vi "Projection View.vi"(6 "Control Ref Queue":T1, 8 "error in (no error)":errorcluster, 11 "3D Plot.lvclass in":refnum<class "3D Plot.lvclass">) -> (0 "error out":errorcluster, 3 "3D Plot.lvclass out":refnum<class "3D Plot.lvclass">)   [LabVIEW 2020, in "3D Plot.lvclass"]
uses:
  3D Plot.lvclass
  3DMathPlot Ctrl Act Queue.ctl
  3DMathPlot Ctrl Act Cluster.ctl
  3DMathPlot State Class.ctl
  3D Plot.lvclass/3D Plot.ctl
  NI_3D Picture Control.lvlib
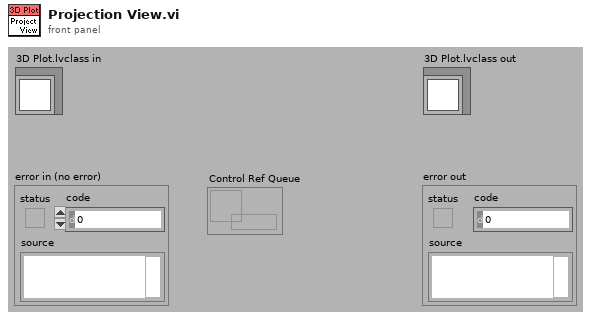
[diagram p1: front panel]
types:
  T1 = typedef "3DMathPlot Ctrl Act Queue.ctl" = refnum<queue>
  T2 = enum32{"Towards X-Y Plane", "Towards X-Z Plane", "Towards Y-Z Plane", "User Defined"}
  T3 = cluster{"View Latitude":sgl, "View Longitude":sgl, "View Distance":sgl}
  T4 = typedef "3DMathPlot Ctrl Act Cluster.ctl" = cluster{"3D Picture Control":refnum<vi>, "Render Window Refnum":refnum<vi>, "XY Graph":refnum<vi>, "Intensity Graph":refnum<vi>, "Color Legend Palette":refnum<vi>, "Projection Palette":refnum<vi>, "XControl  Ref":refnum<vi>, "Facade Ref":refnum<vi>, "Export Image Ref":refnum<vi>, "Clear Data Flag":bool, "Display State Change Class":T5}
  T5 = typedef "3DMathPlot State Class.ctl" = enum16{"Update All Objects (Undo)", "Update Light Object Only", "Update Axis Object Only", "Update Plot Object Only", "Update Cursor Object Only", "Update Axis Plot Cursor Objects", "No Update"}
  T6 = enum16{"None", "Spherical", "Flying", "Oriented"}
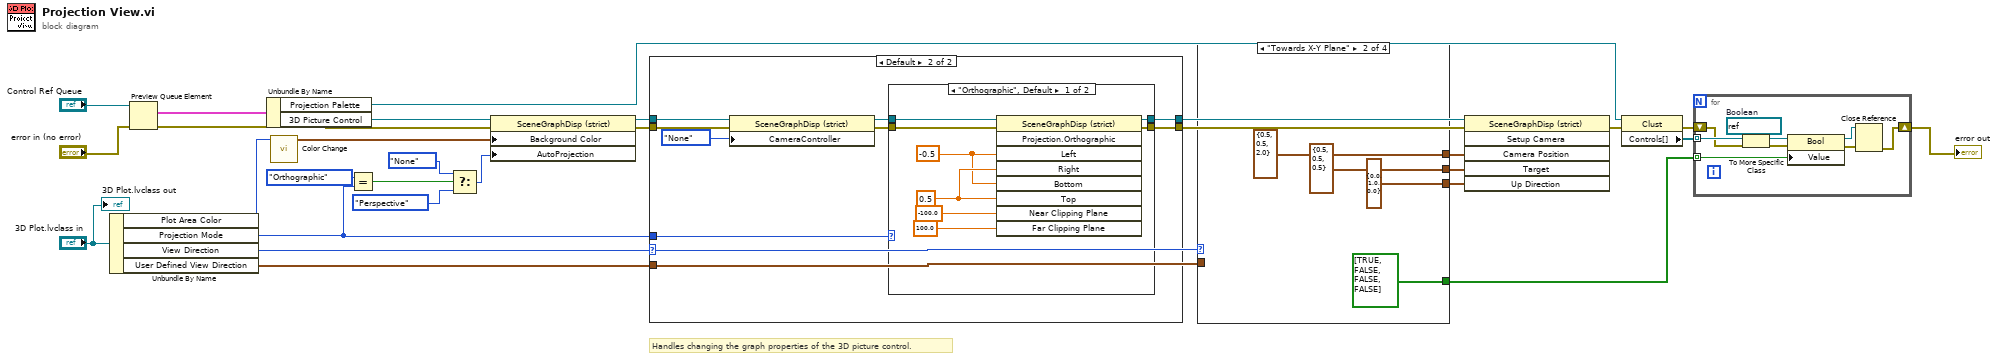
[diagram p0: block diagram]
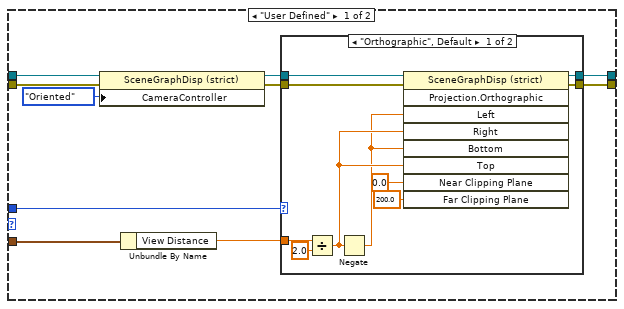
[diagram p2: hidden frame]
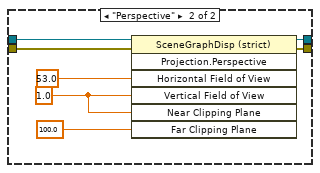
[diagram p4: hidden frame]
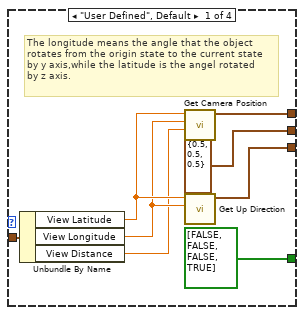
[diagram p5: hidden frame]
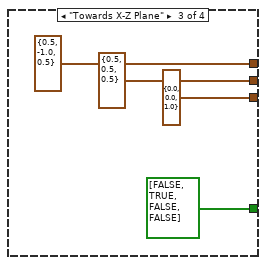
[diagram p6: hidden frame]
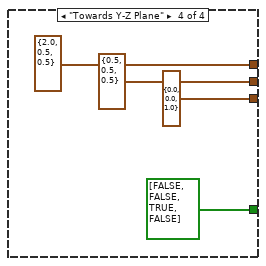
[diagram p7: hidden frame]
diagram:
  # "Handles changing the graph properties of the 3D picture control."
  n1 = Unbundle By Name("3D Plot.lvclass in") -> ("Plot Area Color"=w25:u32, "Projection Mode"=w12:enum16{"Orthographic", "Perspective"}, "View Direction"=w13:T2, "User Defined View Direction"=w11:T3)
  n2 = Preview Queue Element(queue="Control Ref Queue", error in (no error)="error in (no error)") -> (element=w19:T4, error out=w18:errorcluster)  [unwired: 3 out]
  n3 = Unbundle By Name(w19) -> ("Projection Palette"=w5:refnum<vi>, "3D Picture Control"=w20:refnum<vi>)
  n4 = call "Color Change.vi"("Color"=w25) -> ("RGBA"=w21:cluster{"R":sgl, "G":sgl, "B":sgl, "A":sgl})  [unwired: 1 in, 9 out]
  n5 = Equal?(x=enum16{"Orthographic", "Perspective"}."Orthographic" ("y"), y=w12) -> (x = y?=w17:bool)
  n6 = Select(t=enum16{"None", "Perspective", "Orthographic"}."None" ("Automatic Projection Mode"), s=w17, f=enum16{"None", "Perspective", "Orthographic"}."Perspective" ("Automatic Projection Mode")) -> (s? t:f=w14:enum16{"None", "Perspective", "Orthographic"})
  n7 = property class="SceneGraphDisp (strict)"(reference=w20, error in=w18, "Background Color"=w21, "AutoProjection"=w14) -> (reference out=w16:refnum<vi>, error out=w15:errorcluster)
  n8 = case shown="Default" w13 {
    tunnel: w16 -> [w38 w58]
    tunnel: w15 -> [w37 w57]
    tunnel: [w34 w54] -> w9
    tunnel: [w33 w53] -> w10
    tunnel: w12 -> [w32 w52]
    tunnel: w11 -> [w31 _]
    frame "User Defined" {
      n9 = property class="SceneGraphDisp (strict)"(reference=w38, error in=w37, "CameraController"=T6."Oriented" ("Camera Controller:Type")) -> (reference out=w36:refnum<vi>, error out=w35:errorcluster)
      n10 = Unbundle By Name(w31) -> ("View Distance"=w30:sgl)
      n11 = case shown="\"Orthographic\", Default" w32 {
        tunnel: w36 -> [w49 w50]
        tunnel: w35 -> [w48 w51]
        tunnel: [w47 w51] -> w34
        tunnel: [w46 w50] -> w33
        tunnel: w30 -> [w43 _]
        frame "Orthographic", Default {
          n12 = Divide(x=w43, y=sgl 2.0) -> (x/y=w41:sgl)
          n13 = Negate(x=w41) -> (-x=w40:sgl)
          n14 = invoke class="SceneGraphDisp (strict)" method="Projection.Orthographic"(reference=w49, error in=w48, "Left"=w40, "Right"=w41, "Bottom"=w40, "Top"=w41, "Near Clipping Plane"=sgl 0.0, "Far Clipping Plane"=sgl 200.0) -> (reference out=w46:refnum<vi>, error out=w47:errorcluster)  [unwired: 1 in, 7 out]
        }
        frame "Perspective" {
        }
      }
    }
    frame Default {
      n15 = property class="SceneGraphDisp (strict)"(reference=w58, error in=w57, "CameraController"=T6."None" ("Camera Controller:Type")) -> (reference out=w56:refnum<vi>, error out=w55:errorcluster)
      n16 = case shown="\"Orthographic\", Default" w52 {
        tunnel: w56 -> [w67 w72]
        tunnel: w55 -> [w66 w73]
        tunnel: [w65 w74] -> w54
        tunnel: [w62 w69] -> w53
        frame "Orthographic", Default {
          w61 = sgl 0.5 ("Top")
          w60 = sgl -0.5 ("Left")
          n17 = invoke class="SceneGraphDisp (strict)" method="Projection.Orthographic"(reference=w67, error in=w66, "Left"=w60, "Right"=w61, "Bottom"=w60, "Top"=w61, "Near Clipping Plane"=sgl -100.0, "Far Clipping Plane"=sgl 100.0) -> (reference out=w62:refnum<vi>, error out=w65:errorcluster)  [unwired: 1 in, 7 out]
        }
        frame "Perspective" {
          w68 = sgl 1.0 ("Right")
          n18 = invoke class="SceneGraphDisp (strict)" method="Projection.Perspective"(reference=w72, error in=w73, "Horizontal Field of View"=sgl 53.0 ("Left"), "Vertical Field of View"=w68, "Near Clipping Plane"=w68, "Far Clipping Plane"=sgl 100.0 ("Top")) -> (reference out=w69:refnum<vi>, error out=w74:errorcluster)  [unwired: 1 in, 5 out]
        }
      }
    }
  }
  n19 = case shown="\"Towards X-Y Plane\"" w13 {
    tunnel: w11 -> [w82 _ _ _]
    tunnel: [w78 cluster{"X":sgl, "Y":sgl, "Z":sgl} {"X"=0.5, "Y"=0.5, "Z"=2.0} ("Target") cluster{"X":sgl, "Y":sgl, "Z":sgl} {"X"=0.5, "Y"=-1.0, "Z"=0.5} ("Target") cluster{"X":sgl, "Y":sgl, "Z":sgl} {"X"=2.0, "Y"=0.5, "Z"=0.5} ("Target")] -> w8
    tunnel: [cluster{"X":sgl, "Y":sgl, "Z":sgl} {"X"=0.5, "Y"=0.5, "Z"=0.5} ("Target") cluster{"X":sgl, "Y":sgl, "Z":sgl} {"X"=0.5, "Y"=0.5, "Z"=0.5} ("Target") cluster{"X":sgl, "Y":sgl, "Z":sgl} {"X"=0.5, "Y"=0.5, "Z"=0.5} ("Target") cluster{"X":sgl, "Y":sgl, "Z":sgl} {"X"=0.5, "Y"=0.5, "Z"=0.5} ("Target")] -> w7
    tunnel: [w76 cluster{"X":sgl, "Y":sgl, "Z":sgl} {"X"=0.0, "Y"=1.0, "Z"=0.0} ("Target") cluster{"X":sgl, "Y":sgl, "Z":sgl} {"X"=0.0, "Y"=0.0, "Z"=1.0} ("Target") cluster{"X":sgl, "Y":sgl, "Z":sgl} {"X"=0.0, "Y"=0.0, "Z"=1.0} ("Target")] -> w6
    tunnel: [bool[] [FALSE, FALSE, FALSE, TRUE] bool[] [TRUE, FALSE, FALSE, FALSE] bool[] [FALSE, TRUE, FALSE, FALSE] bool[] [FALSE, FALSE, TRUE, FALSE]] -> w1
    frame "User Defined", Default {
      # "The longitude means the angle that the object \nrotates from the origin state to the current state\nby y axis,while the latitude is the angel rotated \nby z axis."
      n20 = Unbundle By Name(w82) -> ("View Latitude"=w81:sgl, "View Longitude"=w80:sgl, "View Distance"=w79:sgl)
      n21 = call "Get Camera Position.vi"("Distance"=w79, "Longitude"=w80, "Latitude"=w81) -> ("Camera Position"=w78:cluster{"X":sgl, "Y":sgl, "Z":sgl})  [unwired: 1 in, 7 out]
      n22 = call "Get Up Direction.vi"("Longitude"=w80, "Latitude"=w81) -> ("Up Direction"=w76:cluster{"X":sgl, "Y":sgl, "Z":sgl})  [unwired: 9 out]
    }
    frame "Towards X-Y Plane" {
    }
    frame "Towards X-Z Plane" {
    }
    frame "Towards Y-Z Plane" {
    }
  }
  n23 = invoke class="SceneGraphDisp (strict)" method="Setup Camera"(reference=w10, error in=w9, "Camera Position"=w8, "Target"=w7, "Up Direction"=w6) -> (error out=w2:errorcluster)  [unwired: 1 in, 5 out]
  n24 = property class="Clust"(reference=w5, error in=w2) -> (error out=w4:errorcluster, "Controls[]"=w3:refnum<vi>[])  [unwired: 1 out]
  n25 = for {
    tunnel: w3 -> [w103] mode=indexing
    shift-right: [w95] -> w29
    shift-left: w4 -> [w100]
    tunnel: w1 -> [w98] mode=indexing
    w101 = refnum<vi> refnum  # Boolean
    n26 = To More Specific Class(target class=w101, reference=w103, error in=w100) -> (specific class reference=w102:refnum<vi>, error out=w99:errorcluster)
    n27 = property class="Bool"(reference=w102, error in=w99, "Value"=w98) -> (reference out=w96:refnum<vi>, error out=w97:errorcluster)
    n28 = Close Reference(reference=w96, error in (no error)=w97) -> (error out=w95:errorcluster)
  }
  "error out" <- w29
  "3D Plot.lvclass out" <- "3D Plot.lvclass in"
